vi "HMI_GetRegPaths.vi"() -> ()   [LabVIEW 2024]
uses:
  Control Definitions/DEF_ConfigRings.ctl
panel:
  out "Array":path[](array[path])
  in  "Test Report":u16(ring) items=["ReportTemplate_03.xlsx", "***Search***"]
  in  "Test Configuration":u16(ring) items=["8005571-05 Elevate OLS .csv", "Level Rig ATP OLS-001 Config1.csv", "Level Rig ATP OLS-001 Config2.csv", "***Search***"]
  in  "Cancel":bool
  in  "OK":bool
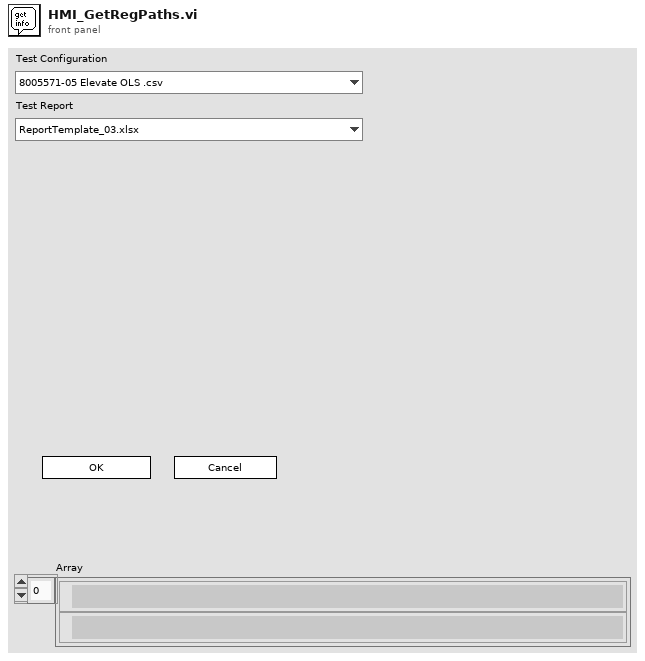
[diagram p1: front panel]
types:
  T1 = typedef "DEF_ConfigRings.ctl" = cluster{"Ring Ctl":refnum<vi>, "Path":path, "Title":string}
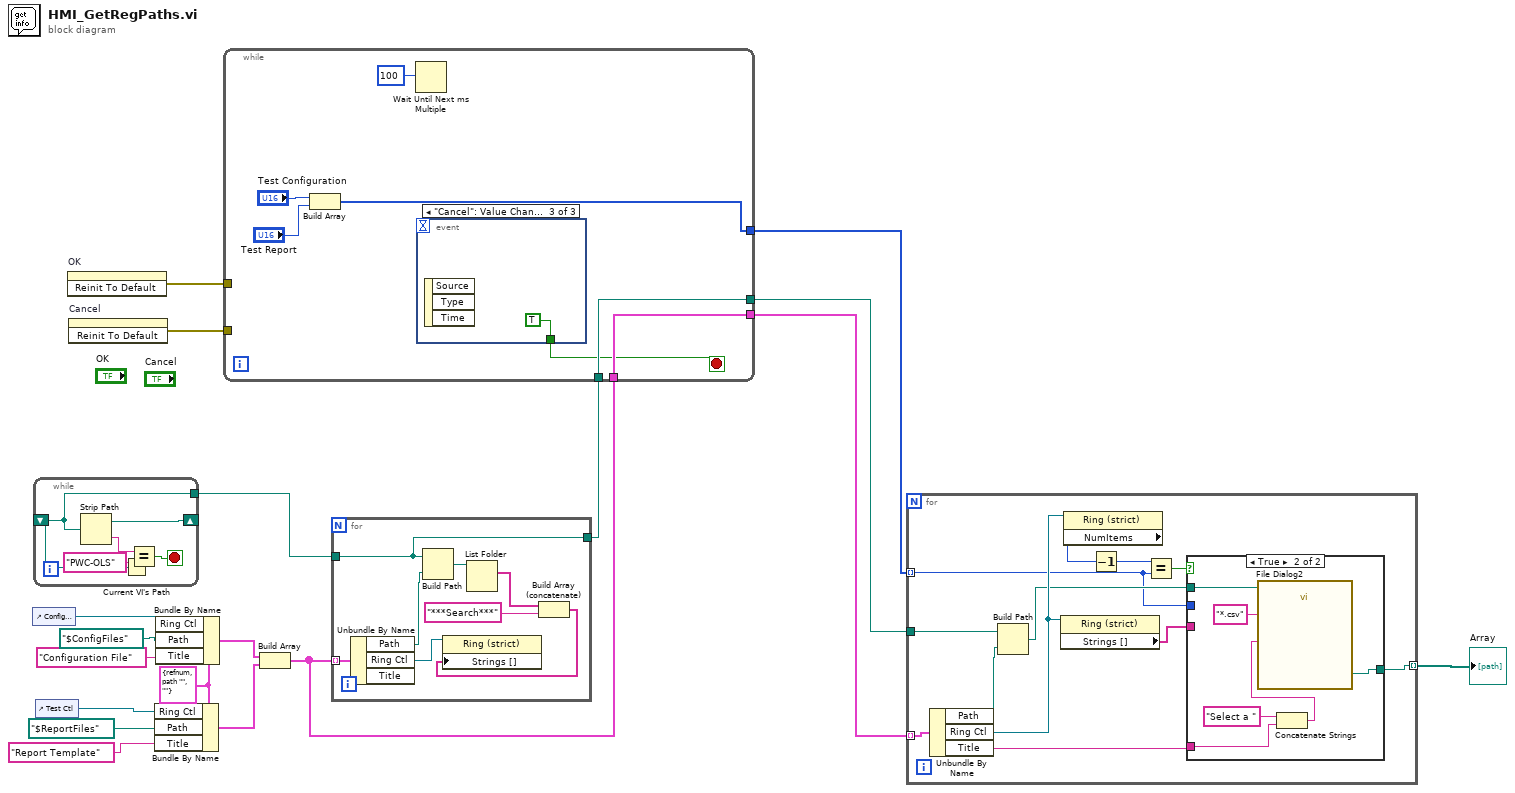
[diagram p0: block diagram]
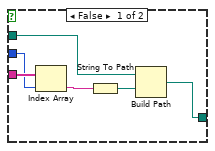
[diagram p2: hidden frame]
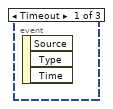
[diagram p3: hidden frame]
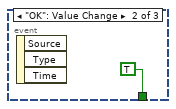
[diagram p4: hidden frame]
diagram:
  w12 = T1 {"Ring Ctl"=refnum, "Path"=path "", "Title"=""} ("output cluster")
  n1 = control-ref of="Config Ctl"() -> (w10:refnum<vi>)
  n2 = control-ref of="Test Ctl"() -> (w14:refnum<vi>)
  n3 = invoke on="OK" class="Bool" method="Reinit To Default"() -> (error out=w19:errorcluster)  [unwired: 3 in, 2 out]
  n4 = invoke on="Cancel" class="Bool" method="Reinit To Default"() -> (error out=w18:errorcluster)  [unwired: 3 in, 2 out]
  n5 = Current VI's Path() -> (path=w17:path)
  n6 = while {
    shift-right: [w24] -> _
    shift-left: w17 -> [w21]
    tunnel: [w21] -> w7
    stop <- w23 stop-if-true
    n7 = Strip Path(path=w21) -> (stripped path=w24:path, name=w20:string)
    n8 = Equal?(x=w20, y="PWC-OLS" ("String")) -> (x = y?=w23:bool)
  }
  n9 = Bundle By Name(cluster=w12, "Ring Ctl"=w14, "Path"=path "$ReportFiles", "Title"="Report Template") -> (w15:T1)
  n10 = Bundle By Name(cluster=w12, "Ring Ctl"=w10, "Path"=path "$ConfigFiles", "Title"="Configuration File") -> (w13:T1)
  n11 = Build Array(w13, w15) -> (w2:T1[])
  n12 = for {
    tunnel: w7 -> [w25]
    tunnel: w2 -> [w28] mode=indexing
    tunnel: [w25] -> w3
    n13 = Unbundle By Name(w28) -> ("Path"=w29:path, "Ring Ctl"=w27:refnum<vi>)  [unwired: 1 out]
    n14 = Build Path(base path=w25, name or relative path=w29) -> (appended path=w26:path)
    n15 = List Folder(path=w26) -> (filenames=w32:string[])  [unwired: 3 in, 3 out]
    n16 = Build Array (concatenate)(w32, "***Search***") -> (w30:string[])
    n17 = property class="Ring (strict)"(reference=w27, "Strings []"=w30) -> ()  [unwired: 1 in, 2 out]
  }
  n18 = while {
    tunnel: w19 -> [_]
    tunnel: w18 -> [_]
    tunnel: [w36] -> w5
    tunnel: [w35] -> w4
    tunnel: w3 -> [w35]
    tunnel: w2 -> [w34]
    tunnel: [w34] -> w1
    stop <- w33 stop-if-true
    n19 = Build Array("Test Configuration", "Test Report") -> (w36:u16[])
    n20 = Wait Until Next ms Multiple(millisecond multiple=100) -> ()  [unwired: 1 out]
    n21 = event shown="[2] \"Cancel\": Value Change" {
      selector: _ -> [_ _ _]
      dyn-events: _ -> [_ _ _]
      timeout: _ -> [_ _ _]
      tunnel: [_ TRUE TRUE] -> w33
      event Timeout {
        n22 = event-data() -> ()  [unwired: 1 in, 3 out]
      }
      event "OK": Value Change {
        n23 = event-data() -> ()  [unwired: 1 in, 3 out]
      }
      event "Cancel": Value Change {
        n24 = event-data() -> ()  [unwired: 1 in, 3 out]
      }
    }
  }
  n25 = for {
    tunnel: w5 -> [w44] mode=indexing
    tunnel: w4 -> [w52]
    tunnel: [w53] -> w6 mode=indexing
    tunnel: w1 -> [w49] mode=indexing
    n26 = Unbundle By Name(w49) -> ("Path"=w50:path, "Ring Ctl"=w48:refnum<vi>, "Title"=w47:string)
    n27 = Build Path(base path=w52, name or relative path=w50) -> (appended path=w46:path)
    n28 = property class="Ring (strict)"(reference=w48) -> ("Strings []"=w45:string[])  [unwired: 1 in, 2 out]
    n29 = property class="Ring (strict)"(reference=w48) -> ("NumItems"=w42:u32)  [unwired: 1 in, 2 out]
    n30 = Decrement(x=w42) -> (x-1=w43:u32)
    n31 = Equal?(x=w43, y=w44) -> (x = y?=w51:bool)
    n32 = case shown="True" w51 {
      tunnel: [w54 w64] -> w53
      tunnel: w46 -> [w55 w63]
      tunnel: w45 -> [w57 _]
      tunnel: w44 -> [w56 _]
      tunnel: w47 -> [_ w61]
      frame False {
        n33 = Index Array(array=w57, index=w56) -> (element=w58:string)
        n34 = String To Path(string=w58) -> (path=w59:path)
        n35 = Build Path(base path=w55, name or relative path=w59) -> (appended path=w54:path)
      }
      frame True {
        n36 = Concatenate Strings("Select a " ("prompt"), w61) -> (w60:string)
        n37 = call "File Dialog2"("start path"=w63, "prompt"=w60, "pattern (all files)"="*.csv" ("default name")) -> ("selected path"=w64:path)  [unwired: 9 in, 3 out]
      }
    }
  }
  "Array" <- w6
